vi "2_24_Fxp_addation.vi"(1 "y":fxp<+/-,24,2>, 2 "x":fxp<+/-,24,2>) -> (0 "x+y":fxp<+/-,25,3> format="%.41g")   [LabVIEW 2020]
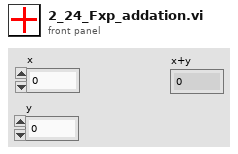
[diagram p1: front panel]
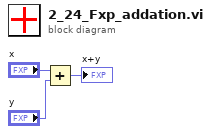
[diagram p0: block diagram]
diagram:
  n1 = Add(x="x", y="y") -> (x+y=→"x+y":fxp<+/-,25,3>)
